vi "SendReply.vi"(0 "reference in":refnum<class "TelegramBOT.lvclass">, 1 "MsgType":T1, 2 "ChatId":i32, 3 "Text":string, 5 "error in (no error)":errorcluster, 9 "ReplyKeyboardMarkup":T2, 11 "reply_to_message_id":i32) -> (14 "reference out":refnum<class "TelegramBOT.lvclass">, 19 "error out":errorcluster)   [LabVIEW 2014, in "TelegramBOT.lvclass"]
uses:
  TelegramBOT.lvclass
  KeyboardMarkup.ctl
  SendMsgType.ctl
  private/SendMessageCluster.ctl
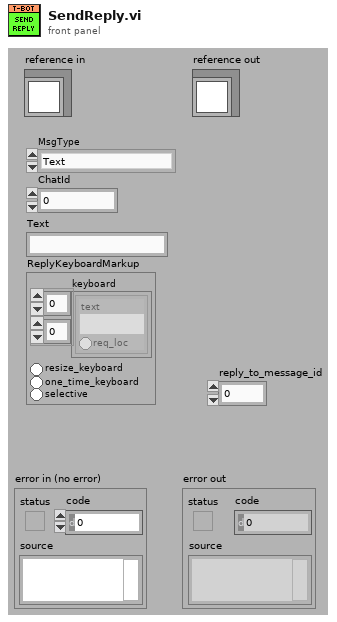
[diagram p1: front panel]
types:
  T1 = typedef "TelegramBOT.lvclass/SendMsgType.ctl" = enum16{"Text", "ReplyKeyboardMarkup", "ReplyKeyboardRemove"}
  T2 = typedef "TelegramBOT.lvclass/KeyboardMarkup.ctl" = cluster{"keyboard":cluster{"text":string, "req_loc":bool}[][], "resize_keyboard":bool, "one_time_keyboard":bool, "selective":bool}
  T3 = typedef "TelegramBOT.lvclass/SendMessageCluster.ctl" = cluster{"chat_id":string, "reply_to_message_id":string, "text":string, "reply_markup":string}
  T4 = cluster{"remove_keyboard":bool, "selective":bool}
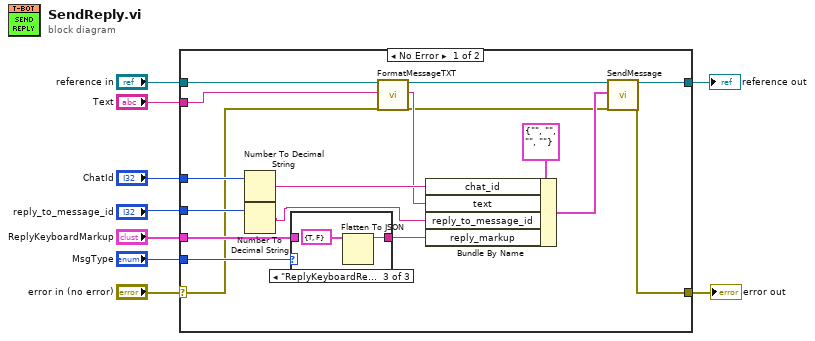
[diagram p0: block diagram]
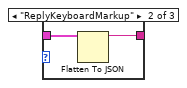
[diagram p3: hidden frame]
diagram:
  n1 = case shown="No Error" "error in (no error)" {
    selector: "error in (no error)" -> [w15 w32]
    tunnel: [w10 w32] -> w8
    tunnel: [w11 w31] -> w6
    tunnel: "reference in" -> [w18 w31]
    tunnel: "Text" -> [w17 _]
    tunnel: "ChatId" -> [w22 _]
    tunnel: "reply_to_message_id" -> [w21 _]
    tunnel: "MsgType" -> [w20 _]
    tunnel: "ReplyKeyboardMarkup" -> [w19 _]
    frame No Error {
      n2 = Number To Decimal String(number=w22) -> (decimal integer string=w26:string)  [unwired: 1 in]
      n3 = Number To Decimal String(number=w21) -> (decimal integer string=w25:string)  [unwired: 1 in]
      n4 = case shown="\"ReplyKeyboardRemove\"" w20 {
        tunnel: [_ w28 w30] -> w23
        tunnel: w19 -> [_ w27 _]
        frame Default {
        }
        frame "ReplyKeyboardMarkup" {
          n5 = Flatten To JSON(anything=w27) -> (JSON string=w28:string)  [unwired: 2 in, 1 out]
        }
        frame "ReplyKeyboardRemove" {
          n6 = Flatten To JSON(anything=T4 {"remove_keyboard"=TRUE, "selective"=FALSE} ("ReplyKeyboardRemove")) -> (JSON string=w30:string)  [unwired: 2 in, 1 out]
        }
      }
      n7 = call "FormatMessageTXT.vi"("reference in"=w18, "Text"=w17, "error in (no error)"=w15) -> ("reference out"=w12:refnum<class "TelegramBOT.lvclass">, "MsgTxt"=w16:string, "error out"=w13:errorcluster)  [unwired: 14 in]
      n8 = Bundle By Name(cluster=T3 {"chat_id"="", "reply_to_message_id"="", "text"="", "reply_markup"=""} ("sendMessage"), "chat_id"=w26, "text"=w16, "reply_to_message_id"=w25, "reply_markup"=w23) -> (w14:T3)
      n9 = call "SendMessage.vi"("reference in"=w12, "sendMessage"=w14, "error in (no error)"=w13) -> ("reference out"=w11:refnum<class "TelegramBOT.lvclass">, "error out"=w10:errorcluster)  [unwired: 15 in]
    }
    frame Error {
    }
  }
  "error out" <- w8
  "reference out" <- w6
